vi "I2C 4 Channel An In ADS1115.vi"() -> ()   [LabVIEW 2020, in "CTI-Scratchpad.lvlib"]
uses:
  CTI-Scratchpad.lvlib
  CTI/Identity.ctl
  CTI-Peripheral/Analog Input/Grove An In/I2C/ADC-ADS1115/Private/ConfigData.ctl
  CTI-Peripheral/Analog Input/Grove An In/I2C/ADC-ADS1115/Private/ADS1115Mode.ctl
  CTI-Peripheral/Analog Input/Grove An In/I2C/ADC-ADS1115/Private/ADS1115Mux.ctl
  CTI-Peripheral/Analog Input/Grove An In/I2C/ADC-ADS1115/Private/ADS1115DataRate.ctl
  CTI-Peripheral/Analog Input/Grove An In/I2C/ADC-ADS1115/Private/ADS1115PGA.ctl
  CTI/Error Reporting.ctl
  CTI/GPIO Number.ctl
  CTI/I2C Number.ctl
  CTI/Session/Session.lvclass
  CTI-Peripheral/Analog Input/Grove An In/I2C/ADC-ADS1115/Grove An In ADS1115.lvclass
  CTI/VisaComms/VisaComms.lvclass
  CTI/CTI.lvlib
panel:
  in  "Configure ADS1115":T1={"Mode"=enum."Single-Shot", "MUX"=enum."Single AI3 - GND", "Data Rate"=enum."8 SPS", "PGA"=enum."FS = ±6.144V"}
  out "Waveform Chart":dbl(graph)
  out "loop":i32
  in  "stop":bool
  out "Identity":T6
  in  "Grove Connector":enum16{"I2C0", "I2C1"}(ring)
  out "error out":errorcluster
  in  "Port":refnum<visa-resource-name>="COM4"
  # "https://wiki.seeedstudio.com/Grove-16-bit-ADC-ADS1115/"
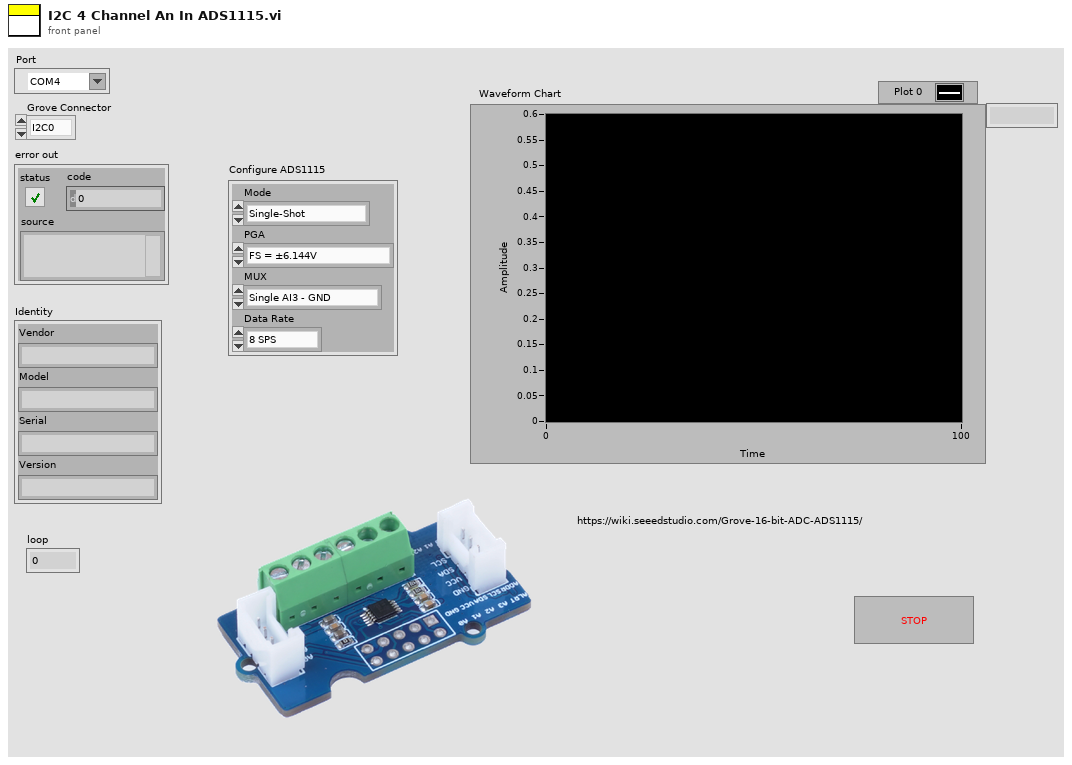
[diagram p1: front panel]
types:
  T1 = typedef "CTI-Peripheral.lvlib/Grove An In ADS1115.lvclass/ConfigData.ctl" = cluster{"Mode":T2, "MUX":T3, "Data Rate":T4, "PGA":T5}
  T2 = typedef "CTI-Peripheral.lvlib/Grove An In ADS1115.lvclass/ADS1115Mode.ctl" = enum16{"Continuous", "Single-Shot"}
  T3 = typedef "CTI-Peripheral.lvlib/Grove An In ADS1115.lvclass/ADS1115Mux.ctl" = enum16{"Single AI0 - GND", "Single AI1 - GND", "Single AI2 - GND", "Single AI3 - GND"}
  T4 = typedef "CTI-Peripheral.lvlib/Grove An In ADS1115.lvclass/ADS1115DataRate.ctl" = enum16{"8 SPS", "16 SPS", "32 SPS", "64 SPS", "128 SPS", "250 SPS", "475 SPS", "860 SPS"}
  T5 = typedef "CTI-Peripheral.lvlib/Grove An In ADS1115.lvclass/ADS1115PGA.ctl" = enum16{"FS = ±6.144V", "FS = ±4.096V", "FS = ±2.048V", "FS = ±1.024V", "FS = ±0.512V", "FS = ±0.256V"}
  T6 = typedef "CTI.lvlib/Identity.ctl" = cluster{"Vendor":string, "Model":string, "Serial":string, "Version":string}
  T7 = typedef "CTI.lvlib/Error Reporting.ctl" = enum16{"Minimal", "Moderate", "Full"}
  T8 = typedef "CTI.lvlib/I2C Number.ctl" = i8
  T9 = typedef "CTI.lvlib/GPIO Number.ctl" = i8
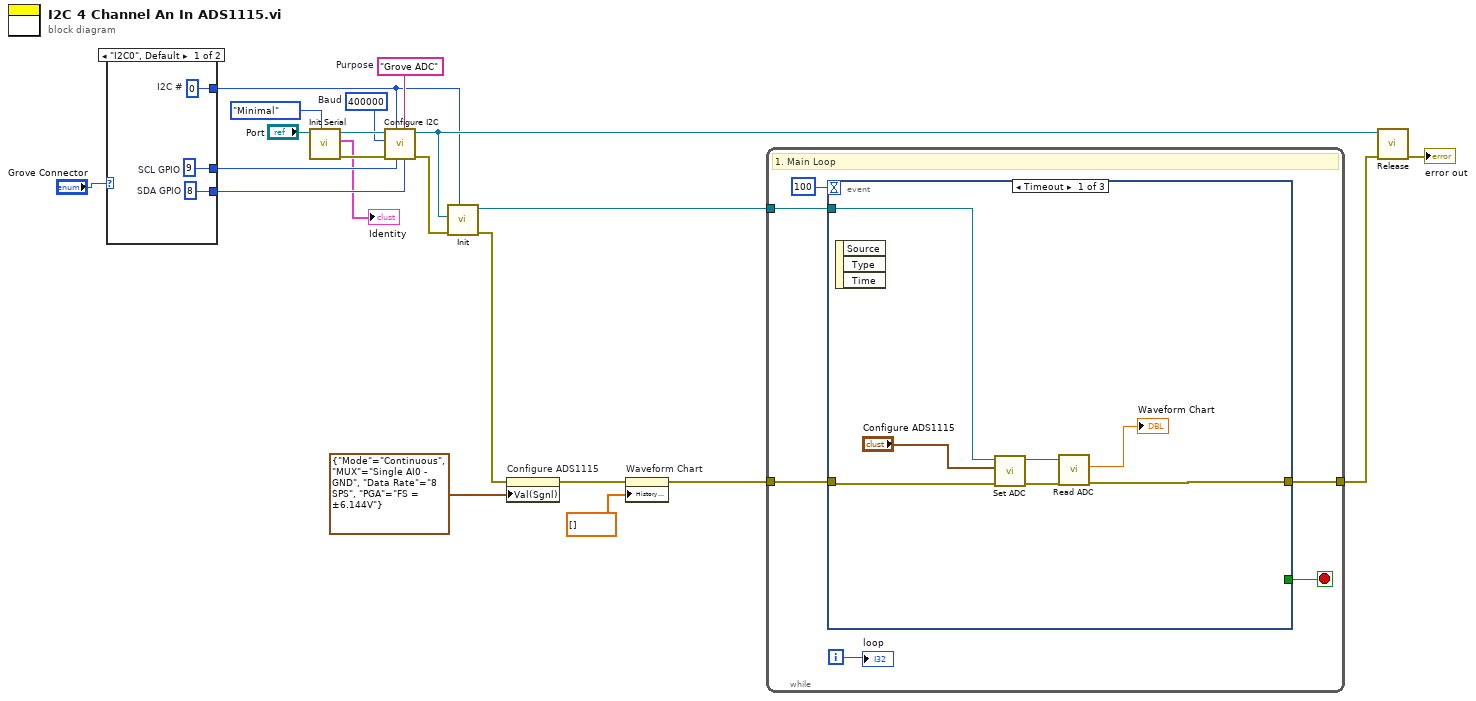
[diagram p0: block diagram]
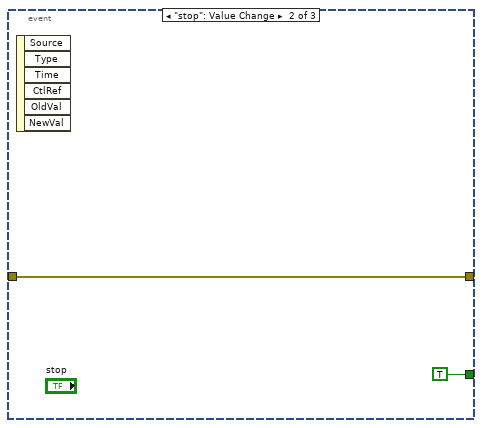
[diagram p2: hidden frame]
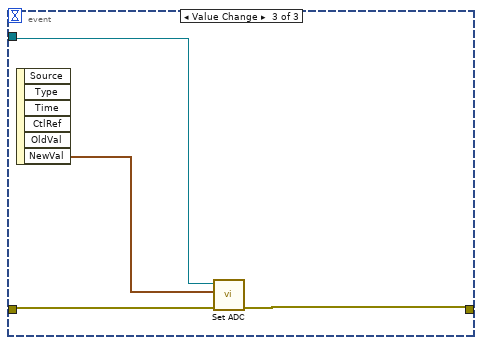
[diagram p3: hidden frame]
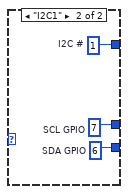
[diagram p4: hidden frame]
diagram:
  w16 = "Grove ADC"  # Purpose
  w17 = u32 400000  # Baud
  n1 = case shown="\"I2C0\", Default" "Grove Connector" {
    tunnel: [w24 w27] -> w12
    tunnel: [w23 w26] -> w11
    tunnel: [w22 w25] -> w10
    frame "I2C0", Default {
      w22 = T8 0  # I2C #
      w23 = T9 8  # SDA GPIO
      w24 = T9 9  # SCL GPIO
    }
    frame "I2C1" {
      w25 = T8 1  # I2C #
      w26 = T9 6  # SDA GPIO
      w27 = T9 7  # SCL GPIO
    }
  }
  n2 = call "Init Serial.vi"("Error Checking (Full)"=Error_Reporting."Minimal", "VISA resource name in"="Port") -> ("error out"=w18:errorcluster, "Identity"=→"Identity":T6, "Session"=w19:refnum<class "Session.lvclass">)  [unwired: 7 in]
  n3 = call "Configure I2C.vi"("SDA GPIO"=w11, "Purpose (\"I2C\")"=w16, "SCL GPIO"=w12, "I2C #"=w10, "error in (no error)"=w18, "Baud"=w17, "Session in"=w19) -> ("error out"=w15:errorcluster, "Session out"=w14:refnum<class "Session.lvclass">)  [unwired: 3 in]
  n4 = call "Init.vi"("I2C #"=w10, "error in (no error)"=w15, "Session In"=w14) -> ("error out"=w5:errorcluster, "ADS115 Out"=w8:refnum<class "Grove An In ADS1115.lvclass">)  [unwired: 7 in]
  n5 = property on="Configure ADS1115" class="Clust (strict)"(error in=w5, "Val(Sgnl)"=T1 {"Mode"=enum."Continuous", "MUX"=enum."Single AI0 - GND", "Data Rate"=enum."8 SPS", "PGA"=enum."FS = ±6.144V"} ("Value (Signaling)")) -> (error out=w3:errorcluster)  [unwired: 1 in, 1 out]
  n6 = property on="Waveform Chart" class="WFChart (strict)"(error in=w3, "History Data"=dbl[] []) -> (error out=w1:errorcluster)  [unwired: 1 in, 1 out]
  n7 = while {
    tunnel: w1 -> [w32]
    tunnel: w8 -> [w33]
    tunnel: [w30] -> w7
    i -> [w31]
    stop <- w28 stop-if-true
    # "1. Main Loop"
    n8 = event shown="[0] Timeout" {
      selector: _ -> [_ _ _]
      dyn-events: _ -> [_ _ _]
      timeout: 100 -> [_ _ _]
      tunnel: w33 -> [w37 _ w44]
      tunnel: w32 -> [w36 w41 w46]
      tunnel: [w40 w41 w43] -> w30
      tunnel: [_ TRUE _] -> w28
      event Timeout {
        n9 = event-data() -> ()  [unwired: 1 in, 3 out]
        n10 = call-dynamic "Set ADC.vi"("error in (no error)"=w36, "Configure ADS1115"="Configure ADS1115", "ADS1115 in"=w37) -> ("error out"=w34:errorcluster, "ADS1115 out"=w38:refnum<class "Grove An In ADS1115.lvclass">)  [unwired: 7 in]
        n11 = call-dynamic "Read ADC.vi"("error in (no error)"=w34, "ADS1115 in"=w38) -> ("error out"=w40:errorcluster, "Data Out"=→"Waveform Chart":dbl)  [unwired: 7 in, 1 out]
      }
      event "stop": Value Change {
        n12 = event-data() -> ()  [unwired: 1 in, 6 out]
      }
      event Value Change {
        n13 = event-data() -> ("NewVal"=w45:T1)  [unwired: 1 in, 5 out]
        n14 = call-dynamic "Set ADC.vi"("error in (no error)"=w46, "Configure ADS1115"=w45, "ADS1115 in"=w44) -> ("error out"=w43:errorcluster)  [unwired: 7 in, 1 out]
      }
    }
    "loop" <- w31
  }
  n15 = call-dynamic "Release.vi"("error in (no error)"=w7, "Session in"=w14) -> ("error out"=→"error out":errorcluster)  [unwired: 9 in]
